vi "BuildPersonnelNameEnum.vi"(8 "error in (no error)":errorcluster) -> (0 "error out":errorcluster, 1 "EnumStringAndVals":cluster{"String":string, "Value":u16}[](array[cluster]), 2 "PUIDs":string[](array[string]), 3 "Roles":T1[](array[typedef]))   [LabVIEW 2015]
uses:
  LVClasses/Personnel/PersonnelType.ctl
  LVClasses/Personnel/Personnel.lvclass/Personnel.ctl
  LVClasses/Personnel/Read Name.vi
  LVClasses/Personnel/Read Role.vi
  LVClasses/Personnel/Read UniqueID.vi
  LVRestAPI/PersonnelRestApi.lvlib
  LVClasses/Personnel/Personnel.lvclass
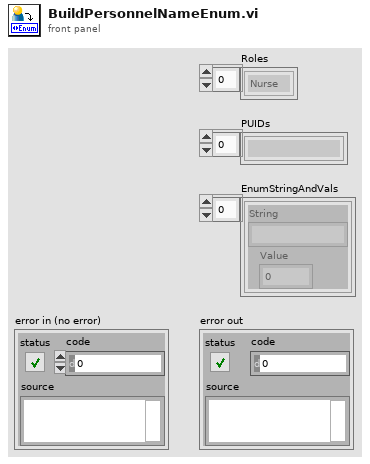
[diagram p1: front panel]
types:
  T1 = typedef "Personnel.lvclass/PersonnelType.ctl" = enum16{"Nurse", "Doctor", "Cleanning", "Admin"}
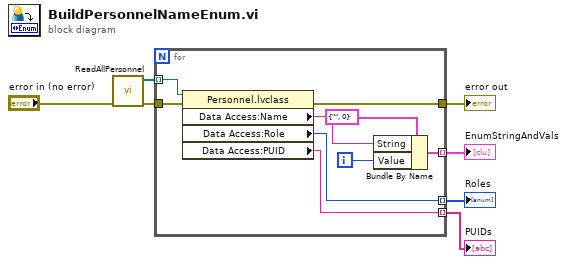
[diagram p0: block diagram]
diagram:
  n1 = call "ReadAllPersonnel.vi"("error in (no error)"="error in (no error)") -> ("error out"=w3:errorcluster, "Personnel"=w2:refnum<class "Personnel.lvclass">[])  [unwired: 7 in, 2 out]
  n2 = for {
    tunnel: w2 -> [w16] mode=indexing
    tunnel: w3 -> [w15]
    tunnel: [w14] -> w4
    tunnel: [w13] -> w5 mode=indexing
    tunnel: [w10] -> w6 mode=indexing
    tunnel: [w8] -> w7 mode=indexing
    i -> [w11]
    n3 = property class="Personnel.lvclass"(reference=w16, error in=w15) -> (error out=w14:errorcluster, "Data Access:Name"=w9:string, "Data Access:Role"=w10:T1, "Data Access:PUID"=w8:string)  [unwired: 1 out]
    n4 = Bundle By Name(cluster=cluster{"String":string, "Value":u16} {"String"="", "Value"=0}, "String"=w9, "Value"=w11) -> (w13:cluster{"String":string, "Value":u16})
  }
  "PUIDs" <- w7
  "Roles" <- w6
  "EnumStringAndVals" <- w5
  "error out" <- w4
